vi "Read (SubVI).vi"(8 "error in (no error)":errorcluster, 11 "Parameter In":T1={"ReadIntParam"=TRUE, "ReadDescrParam"=FALSE, "ReadFloatParam"=TRUE, "debug"=FALSE, "ReadJSON"=TRUE, "IP_address"="192.168.1.216", "N_attempts"=3, "type_con"=enum."TCP", "MB_address"=1, "VISA"="COM1", "connection ID"=refnum, "nameDevices"="", "timeout"=3000, "port"=2000, "type_version"="0F0C0001", "baud_rate"=115200, "VersionControl"=TRUE, "TCP_conn"=TRUE, "WindowSize"=700}) -> (0 "error out":errorcluster, 1 "String out":string, 3 "Parameter Out":T1={"ReadIntParam"=TRUE, "ReadDescrParam"=FALSE, "ReadFloatParam"=TRUE, "debug"=FALSE, "ReadJSON"=TRUE, "IP_address"="192.168.1.216", "N_attempts"=3, "type_con"=enum."TCP", "MB_address"=1, "VISA"="COM1", "connection ID"=refnum, "nameDevices"="", "timeout"=3000, "port"=2000, "type_version"="0F0C0001", "baud_rate"=115200, "VersionControl"=TRUE, "TCP_conn"=TRUE, "WindowSize"=700}, 5 "ErrorMessage":bool, 7 "GatewayTimeout":bool)   [LabVIEW 2017, in "LV_Unicorn.lvlib"]
uses:
  LV_Unicorn.lvlib
  Control/unicorn_conn.ctl
panel:
  out "MessageReceived":bool
  out "Attempts":i32
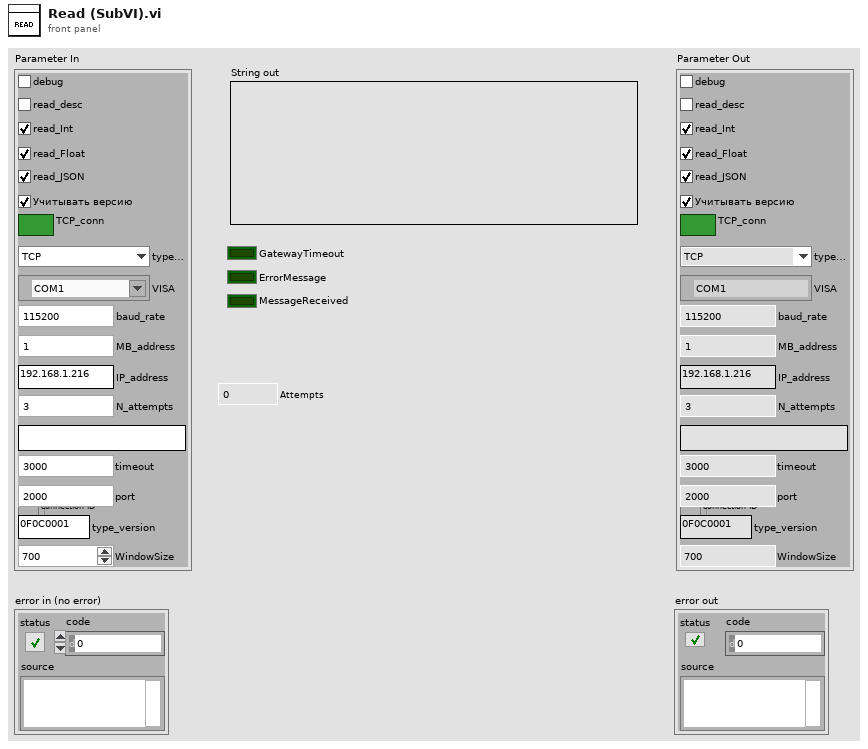
[diagram p1: front panel]
types:
  T1 = typedef "LV_Unicorn.lvlib/unicorn_conn.ctl" = cluster{"ReadIntParam":bool, "ReadDescrParam":bool, "ReadFloatParam":bool, "debug":bool, "ReadJSON":bool, "IP_address":string, "N_attempts":i32, "type_con":enum16{"Serial", "TCP"}, "MB_address":i32, "VISA":refnum<visa-resource-name>, "connection ID":refnum<k5>, "nameDevices":string, "timeout":i32, "port":u16, "type_version":string, "baud_rate":u32, "VersionControl":bool, "TCP_conn":bool, "WindowSize":i32}
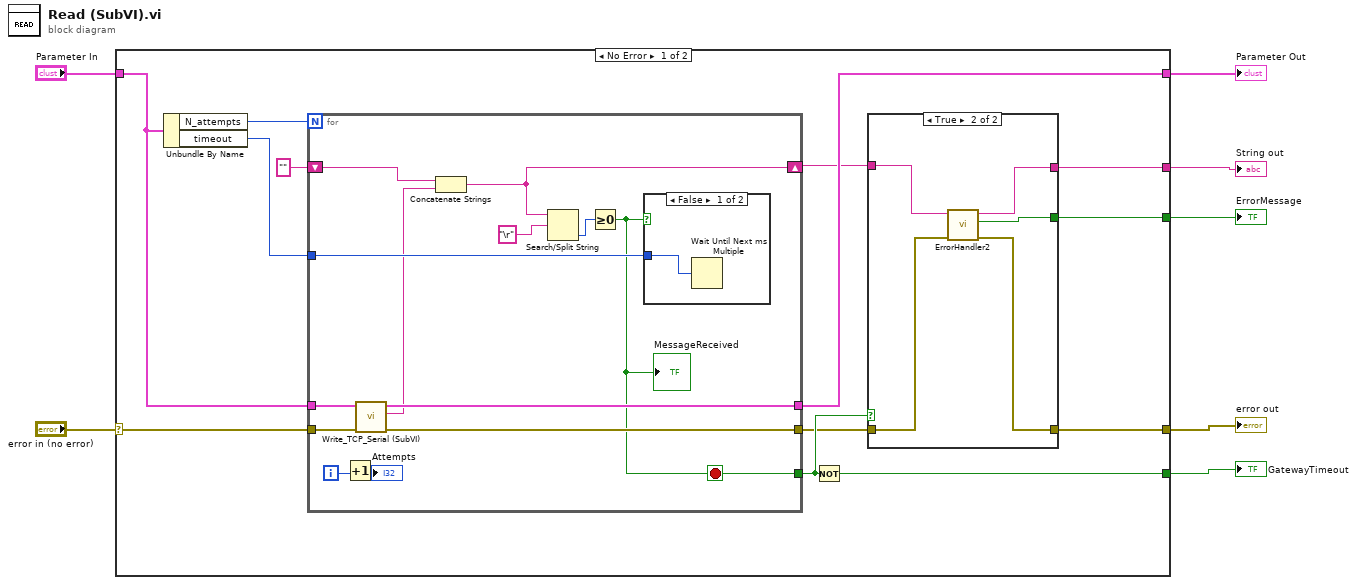
[diagram p0: block diagram]
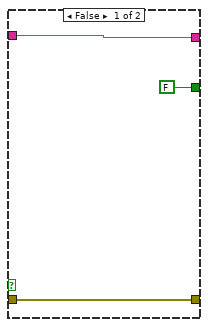
[diagram p2: hidden frame]
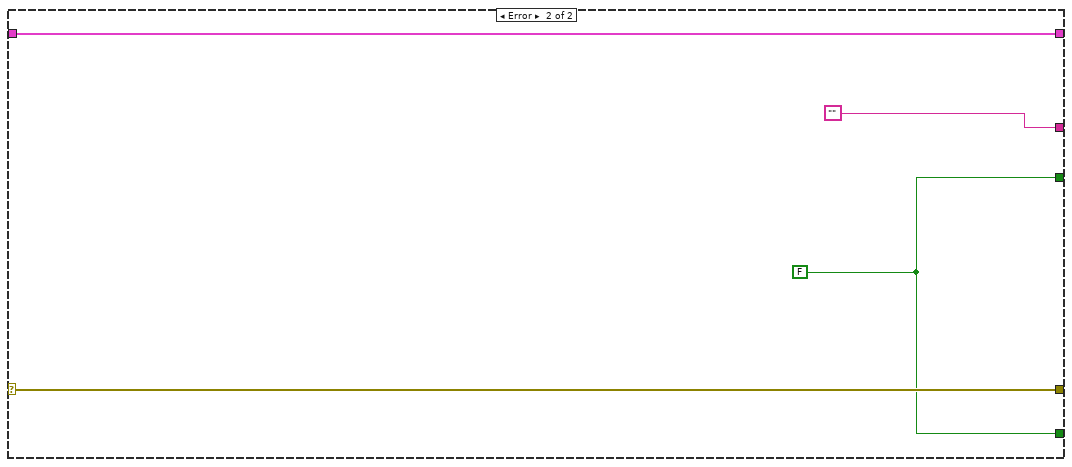
[diagram p4: hidden frame]
diagram:
  n1 = case shown="No Error" "error in (no error)" {
    selector: "error in (no error)" -> [w18 w44]
    tunnel: [w9 w44] -> w7
    tunnel: "Parameter In" -> [w20 w45]
    tunnel: [w19 w45] -> w5
    tunnel: [w11 ""] -> w3
    tunnel: [w14 w42] -> w2
    tunnel: [w8 w42] -> w1
    frame No Error {
      n2 = Unbundle By Name(w20) -> ("N_attempts"=w16:i32, "timeout"=w15:i32)
      n3 = for {
        N: w16 -> [_]
        tunnel: [w35] -> w10
        tunnel: w18 -> [w40]
        shift-right: [w34] -> w12
        shift-left: "" ("read buffer") -> [w39]
        tunnel: w15 -> [w38]
        tunnel: w20 -> [w37]
        tunnel: [w36] -> w19
        tunnel: [w29] -> w13
        i -> [w30]
        stop <- w29 stop-if-true
        n4 = Increment(x=w30) -> ()  [unwired: 1 out]
        n5 = call "Write_TCP_Serial (SubVI).vi"("error in (no error)"=w40, "connectionParamIn"=w37) -> ("error out"=w35:errorcluster, "data out"=w31:string, "connectionParamOut"=w36:T1)  [unwired: 7 in]
        n6 = Concatenate Strings(w39, w31) -> (w34:string)
        n7 = Search/Split String(string=w34, search string/char (-)="\r") -> (offset of match=w32:i32)  [unwired: 1 in, 2 out]
        n8 = Greater Or Equal To 0?(x=w32) -> (x >= 0?=w29:bool)
        "MessageReceived" <- w29
        n9 = case shown="False" w29 {
          tunnel: w38 -> [w41 _]
          frame False {
            n10 = Wait Until Next ms Multiple(millisecond multiple=w41) -> ()  [unwired: 1 out]
          }
          frame True {
          }
        }
      }
      n11 = Not(x=w13) -> (.not. x?=w14:bool)
      n12 = case shown="True" w13 {
        tunnel: w12 -> [w23 w28]
        tunnel: [w23 w24] -> w11
        tunnel: w10 -> [w22 w27]
        tunnel: [w22 w26] -> w9
        tunnel: [FALSE ("ErrorMessage") w25] -> w8
        frame False {
        }
        frame True {
          n13 = call "ErrorHandler2.vi"("error in"=w27, "StringIn"=w28) -> ("output cluster"=w26:errorcluster, "ErrorMessage"=w25:bool, "StringOut"=w24:string)  [unwired: 7 in]
        }
      }
    }
    frame Error {
      w42 = FALSE ("Ошибка пакета?")
    }
  }
  "error out" <- w7
  "Parameter Out" <- w5
  "String out" <- w3
  "ErrorMessage" <- w1
  "GatewayTimeout" <- w2
